vi "getFieldTypes.vi"(8 "error in (no error)":errorcluster, 11 "IStructType in":refnum<class "IStructType.lvclass">) -> (0 "error out":errorcluster, 2 "Field Types out":refnum<class "IType.lvclass">[](array[class]), 3 "IStructType out":refnum<class "IStructType.lvclass">)   [LabVIEW 2022 SP3, in "openDAQ.lvlib" / "daqCoreTypes.lvlib" / "IStructType.lvclass"]
uses:
  <instrlib>/openDAQ/Public/Classes/daqCoreTypes/IStructType/IStructType.lvclass
  <instrlib>/openDAQ/Public/Classes/daqCoreTypes/IStructType/IStructType.lvclass/IStructType.ctl
  <instrlib>/openDAQ/Public/Classes/daqCoreTypes/IList/IList.lvclass
  <instrlib>/openDAQ/Binaries/Windows/x86/copendaq32.dll
  <instrlib>/openDAQ/Public/Classes/daqCoreTypes/IList/Polymorphic/getList/getTypeList.vi
  <instrlib>/openDAQ/Public/Classes/IType/IType.lvclass
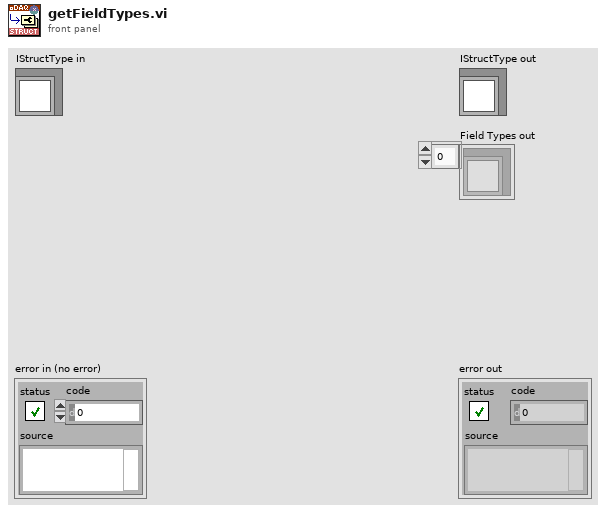
[diagram p1: front panel]
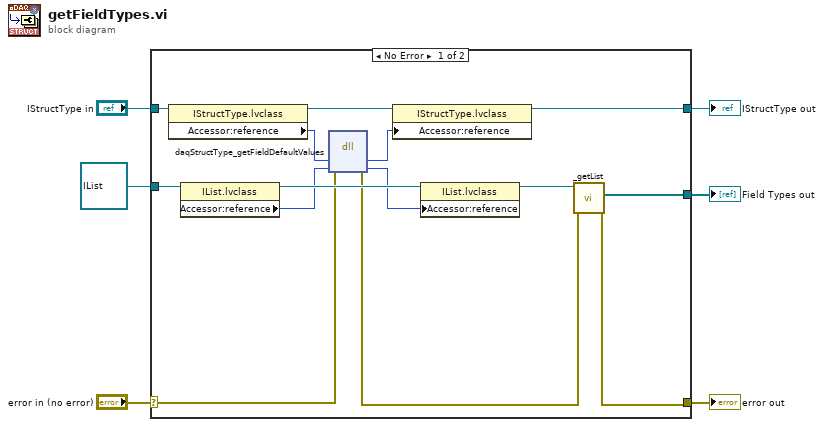
[diagram p0: block diagram]
diagram:
  n1 = case shown="No Error" "error in (no error)" {
    selector: "error in (no error)" -> [w11 w22]
    tunnel: [w7 w22] -> w5
    tunnel: [w18 w21] -> w3
    tunnel: "IStructType in" -> [w19 w21]
    tunnel: refnum<class "IList.lvclass"> refnum ("openDAQ.lvlib:daqCoreTypes.lvlib:IList.lvclass") -> [w14 _]
    tunnel: [w9 _] -> w1
    frame No Error {
      n2 = property class="IStructType.lvclass"(reference=w19) -> (reference out=w17:refnum<class "IStructType.lvclass">, "Accessor:reference"=w16:i64)  [unwired: 1 in, 1 out]
      n3 = property class="IList.lvclass"(reference=w14) -> (reference out=w20:refnum<class "IList.lvclass">, "Accessor:reference"=w13:i64)  [unwired: 1 in, 1 out]
      n4 = dll-call lib="C:/Program Files (x86)/National Instruments/LabVIEW 2022/instr.lib/openDAQ/Binaries/Windows/x86/copendaq*.*" fn="daqStructType_getFieldDefaultValues"(error in=w11, "type"=w16, "values"=w13) -> (error out=w8:errorcluster, "type"=w15:i64, "values"=w12:i64)  [unwired: 3 in, 1 out]
      n5 = property class="IStructType.lvclass"(reference=w17, "Accessor:reference"=w15) -> (reference out=w18:refnum<class "IStructType.lvclass">)  [unwired: 1 in, 1 out]
      n6 = property class="IList.lvclass"(reference=w20, "Accessor:reference"=w12) -> (reference out=w10:refnum<class "IList.lvclass">)  [unwired: 1 in, 1 out]
      n7 = call-poly <instrlib>:"_getList.vi"("error in (no error)"=w8, "IList in"=w10) -> ("error out"=w7:errorcluster, "baseObjects out"=w9:refnum<class "IType.lvclass">[])  [unwired: 8 in]
    }
    frame Error {
    }
  }
  "error out" <- w5
  "IStructType out" <- w3
  "Field Types out" <- w1
